vi "Get region dimensions - SubVI.vi"(11 "x1y1x2y2":u16[](array[numeric])) -> (0 "y size":u64=1024, 1 "x size":u64=1024, 2 "y origin":u64, 3 "x origin":u64)   [LabVIEW 2014]
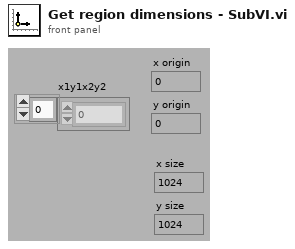
[diagram p1: front panel]
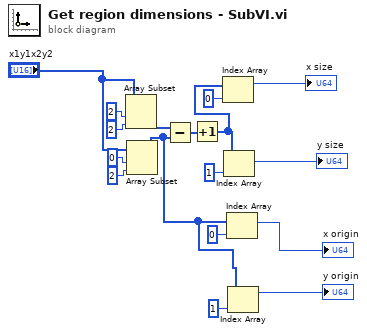
[diagram p0: block diagram]
diagram:
  n1 = Array Subset(array="x1y1x2y2", index=2, length=2) -> (w13:u16[])
  n2 = Array Subset(array="x1y1x2y2", index=0, length=2) -> (w3:u16[])
  n3 = Subtract(x=w13, y=w3) -> (x-y=w14:u16[])
  n4 = Increment(x=w14) -> (x+1=w15:u16[])
  n5 = Index Array(array=w15, index=0) -> (element=→"x size":u16)
  n6 = Index Array(array=w15, index=1) -> (element=→"y size":u16)
  n7 = Index Array(array=w3, index=0) -> (element=→"x origin":u16)
  n8 = Index Array(array=w3, index=1) -> (element=→"y origin":u16)
